vi "Set Server Internal UEs.vi"(10 "Server Internal UEs":T1, 11 "OOP Server in":refnum<class "HVC.lvclass">) -> (3 "OOP Server out":refnum<class "HVC.lvclass">)   [LabVIEW 2019, in "HVC.lvlib" / "HVC.lvclass"]
uses:
  HVC.lvclass
  typeDefs/Server Internal UEs.ctl
  typeDefs/Server Internal Message.ctl
  HVC.lvclass/HVC.ctl
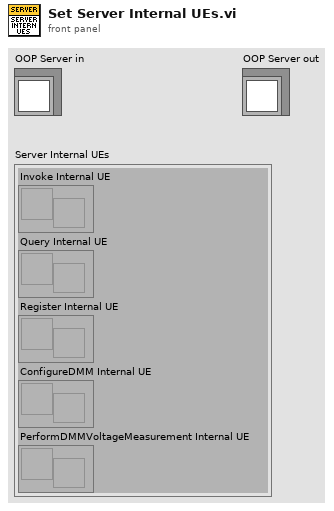
[diagram p1: front panel]
types:
  T1 = typedef "HVC.lvlib/HVC.lvclass/Server Internal UEs.ctl" = cluster{"Invoke Internal UE":refnum<user-event>, "Query Internal UE":refnum<user-event>, "Register Internal UE":refnum<user-event>, "ConfigureDMM Internal UE":refnum<user-event>, "PerformDMMVoltageMeasurement Internal UE":refnum<user-event>}
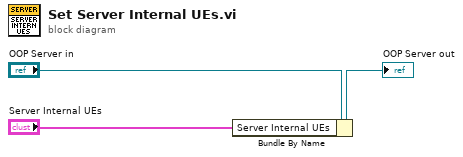
[diagram p0: block diagram]
diagram:
  n1 = Bundle By Name(cluster="OOP Server in", "Server Internal UEs"="Server Internal UEs") -> (→"OOP Server out":refnum<class "HVC.lvclass">)
